vi "XY Graph Smoothen Multiple Plots (Cubic Spline).vi"(6 "balance parameter (-1: auto)":dbl=-1.0, 8 "error in (no error)":errorcluster, 9 "Tail only (F)":bool, 10 "Selected Plots":i32[](array[numeric]), 11 "Selected Plot Info":T1) -> (0 "error out":errorcluster, 1 "Smoothened Plot Message":string, 3 "Last Smoothened Plot":cluster{"t Array":dbl[], "IRF Array":dbl[]}, 4 "Single Plot?":bool)   [LabVIEW 2021, in "XY Graph Add-Ons.lvlib"]
uses:
  XY Graph Add-Ons.lvlib
  XY Graph Selected Plot Info.ctl
  XY Graph Refnum.ctl
  <vilib>/Utility/miscctls.llb/LVPoint32TypeDef.ctl
  Strings/Strings.lvlib
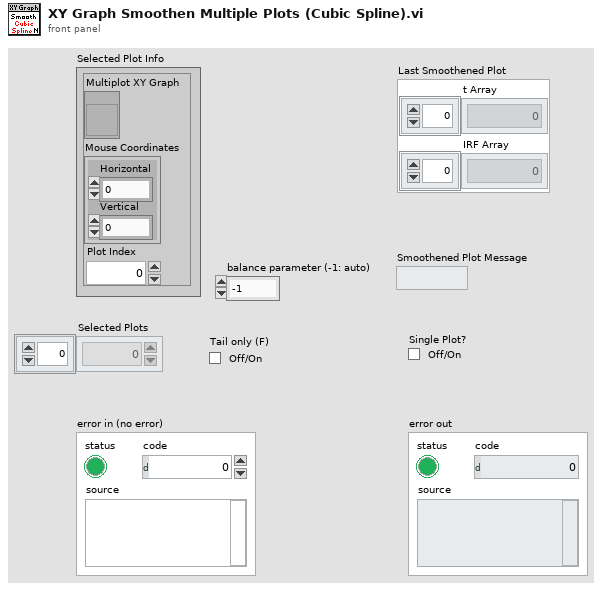
[diagram p1: front panel]
types:
  T1 = typedef "XY Graph Add-Ons.lvlib/XY Graph Selected Plot Info.ctl" = cluster{"Multiplot XY Graph":T2, "Mouse Coordinates":T3, "Plot Index":i32}
  T2 = typedef "XY Graph Add-Ons.lvlib/XY Graph Refnum.ctl" = refnum<vi>
  T3 = typedef "LVPoint32TypeDef.ctl" = cluster{"Horizontal":i32, "Vertical":i32}
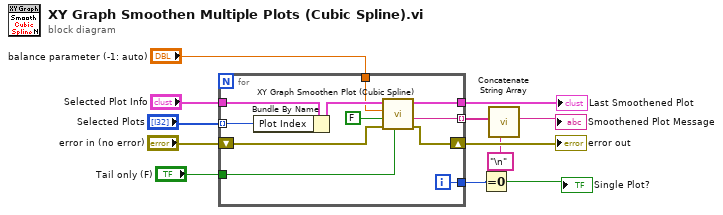
[diagram p0: block diagram]
diagram:
  n1 = for {
    tunnel: "Selected Plot Info" -> [w23]
    tunnel: [w21] -> w7 mode=indexing
    tunnel: [w19] -> w9
    shift-right: [w20] -> w10
    shift-left: "error in (no error)" -> [w22]
    tunnel: "Selected Plots" -> [w17] mode=indexing
    tunnel: [w16] -> w4
    tunnel: "Tail only (F)" -> [w14]
    tunnel: "balance parameter (-1: auto)" -> [w13]
    i -> [w16]
    n2 = Bundle By Name(cluster=w23, "Plot Index"=w17) -> (w18:T1)
    n3 = call "XY Graph Smoothen Plot (Cubic Spline).vi"("Tail only (F)"=w14, "error in (no error)"=w22, "Replace Plot (T)?"=FALSE, "balance parameter (-1: auto)"=w13, "Selected Plot Info"=w18) -> ("Error Out"=w20:errorcluster, "Smooth Plot Message"=w21:string, "Smoothed Plot"=w19:cluster{"X Array":dbl[], "Y Array":dbl[]})  [unwired: 4 in]
  }
  "error out" <- w10
  "Last Smoothened Plot" <- w9
  n4 = Equal To 0?(x=w4) -> (x = 0?=→"Single Plot?":bool)
  n5 = call "Concatenate String Array.vi"("Separator (TAB)"="\n", "String Array"=w7) -> ("Formatted String"=→"Smoothened Plot Message":string)  [unwired: 9 in]
